vi "FormulaNode.vi"() -> ()   [LabVIEW 2020]
panel:
  out "output variable":dbl
  in  "Cateto2":dbl
  in  "Cateto1":dbl
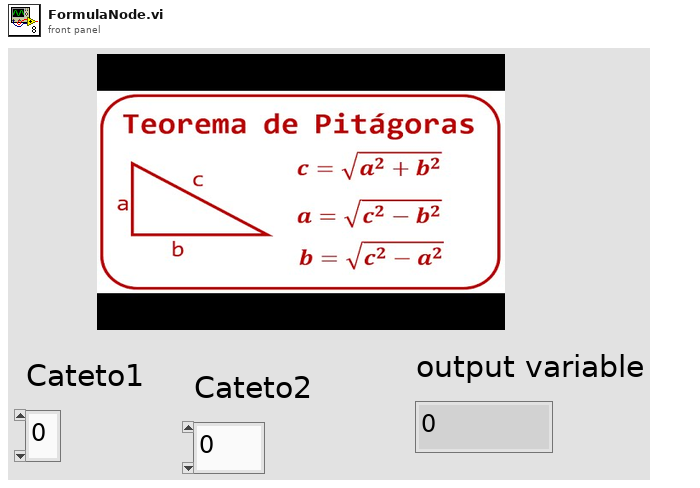
[diagram p1: front panel]
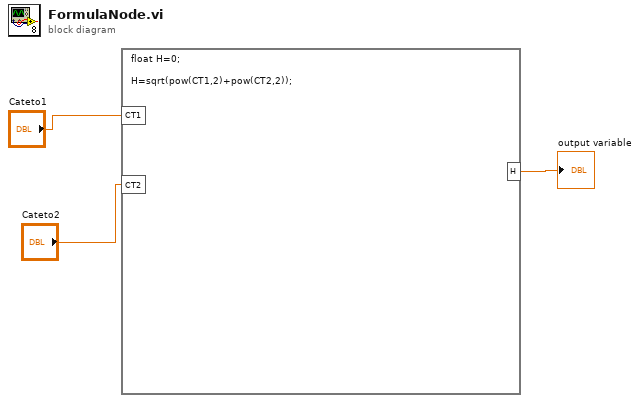
[diagram p0: block diagram]
diagram:
  n1 = formula code="float H=0;\n\nH=sqrt(pow(CT1,2)+pow(CT2,2));"("CT1"="Cateto1", "CT2"="Cateto2") -> ("H"=→"output variable":dbl)
